vi "DatabaseHand_is_queue.vi"(8 "error in (no error)":errorcluster, 10 "name":string, 11 "Database RefNum in":T1) -> (0 "error out":errorcluster, 2 "queue?":bool, 3 "Database RefNum out":T1)   [LabVIEW 2016]
uses:
  private/vis/DatabaseHand_RefNum.ctl
  private/vis/DatabaseHand_Element_Get(string).vi
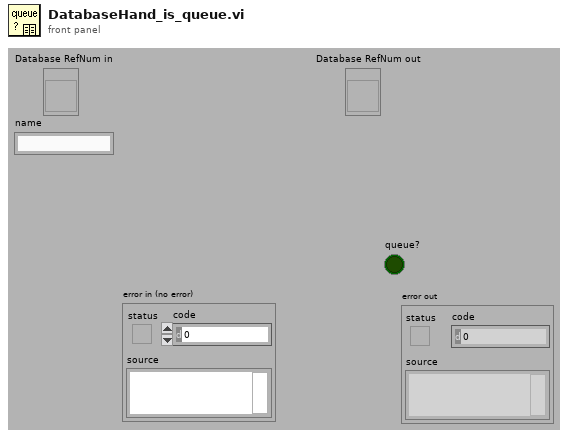
[diagram p1: front panel]
types:
  T1 = typedef "DatabaseHand_RefNum.ctl" = refnum<vi>
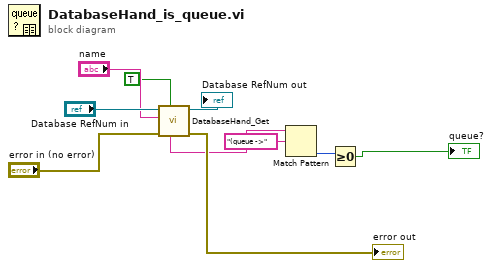
[diagram p0: block diagram]
diagram:
  n1 = call-poly "DatabaseHand_Get.vi"("nd queue"=TRUE, "error in (no error)"="error in (no error)", "name"="name", "Database RefNum in"="Database RefNum in") -> ("error out"=→"error out":errorcluster, "Database RefNum out"=→"Database RefNum out":T1, "unit"=w3:string)  [unwired: 1 in, 4 out]
  n2 = Match Pattern(string=w3, regular expression="(queue ->") -> (offset past match=w4:i32)  [unwired: 4 out]
  n3 = Greater Or Equal To 0?(x=w4) -> (x >= 0?=→"queue?":bool)
